vi "Write.vi"(6 "wait for reply (T)":bool=TRUE, 8 "error in (no error)":errorcluster, 10 "Command":string) -> (0 "error out":errorcluster, 1 "timed out?":bool, 2 "Reply Payload":T1)   [LabVIEW 2017, in "FingerPrintMânager.lvlib"]
doc: "_____\nCreated using Delacor QMH Event Scripter 4.1.0.80."
uses:
  Write (Reply Payload)--cluster.ctl
  Write Argument--cluster.ctl
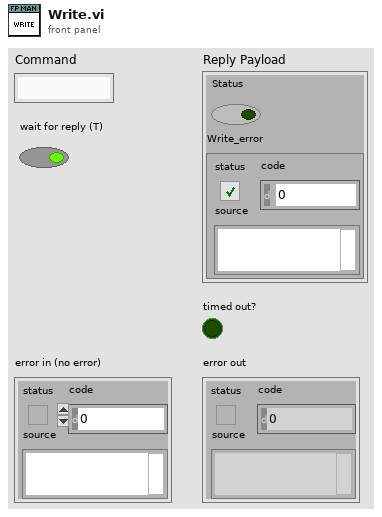
[diagram p1: front panel]
types:
  T1 = typedef "FingerPrintMânager.lvlib/Write (Reply Payload)--cluster.ctl" = cluster{"Status":bool, "Write_error":errorcluster}
  T2 = typedef "FingerPrintMânager.lvlib/Write Argument--cluster.ctl" = cluster{"Command":string, "Wait Notifier":refnum<notifier>, "wait for reply":bool}
  T3 = typedef "FingerPrintMânager.lvlib/Request Events--cluster.ctl" = cluster{"Stop Module":refnum<user-event>, "Show Panel":refnum<user-event>, "Hide Panel":refnum<user-event>, "Get Module Execution Status":refnum<user-event>, "Show Diagram":refnum<user-event>, "Init":refnum<user-event>, "UnInit":refnum<user-event>, "Write":refnum<user-event>, "Read":refnum<user-event>, "UpdatePump":refnum<user-event>, "StopPump":refnum<user-event>}
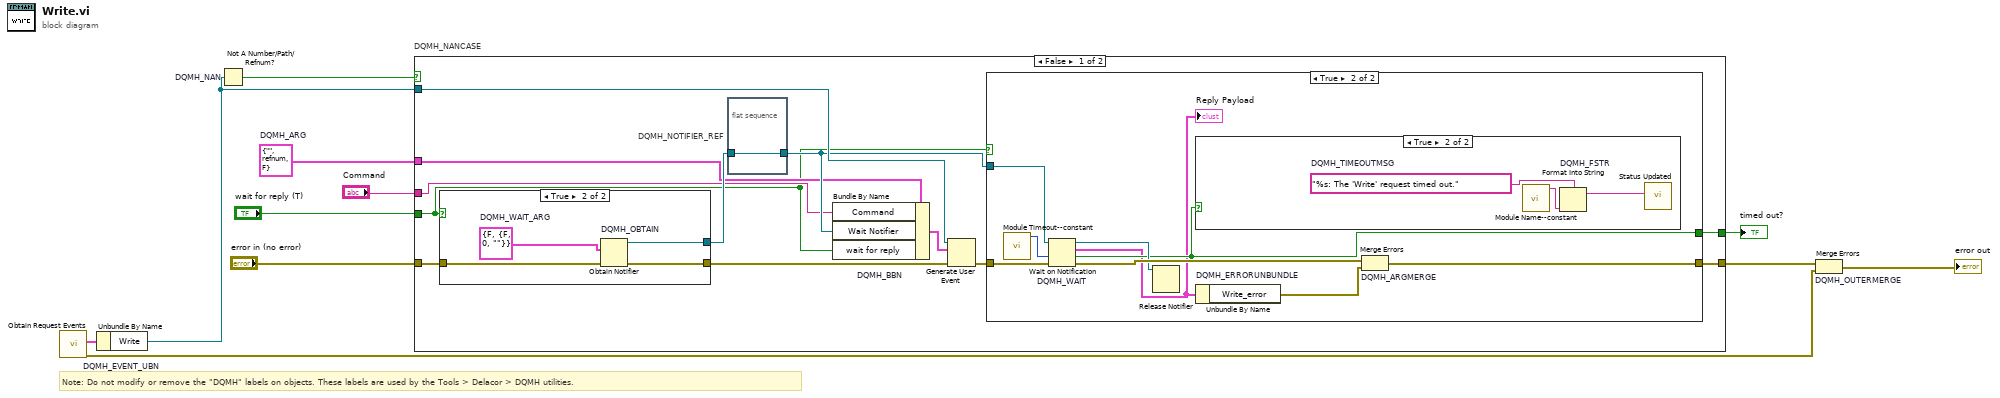
[diagram p0: block diagram]
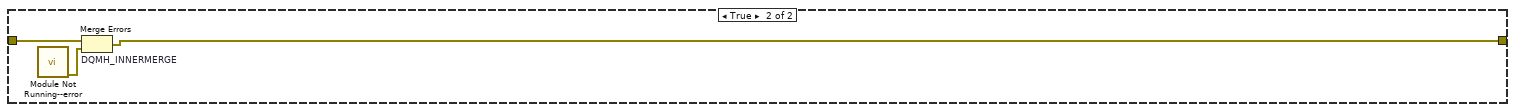
[diagram p5: hidden frame]
diagram:
  w5 = T2 {"Command"="", "Wait Notifier"=refnum, "wait for reply"=FALSE}  # DQMH_ARG
  # "Note: Do not modify or remove the \"DQMH\" labels on objects. These labels are used by the Tools > Delacor > DQMH utilities."
  n1 = call "Obtain Request Events.vi"() -> ("error out"=w2:errorcluster, "FingerPrintMânager Request Events"=w1:T3)  [unwired: 10 in]
  n2 = Unbundle By Name "DQMH_EVENT_UBN"(w1) -> ("Write"=w9:refnum<user-event>)
  n3 = Not A Number/Path/Refnum? "DQMH_NAN"(number/path/refnum=w9) -> (NaN/Path/Refnum?=w8:bool)
  n4 = case "DQMH_NANCASE" shown="False" w8 {
    tunnel: "error in (no error)" -> [w23 w45]
    tunnel: w9 -> [w21 _]
    tunnel: [w18 w44] -> w6
    tunnel: [w19 _] -> w7
    tunnel: w5 -> [w14 _]
    tunnel: "Command" -> [w13 _]
    tunnel: "wait for reply (T)" -> [w12 _]
    frame False {
      n5 = case shown="True" w12 {
        tunnel: w23 -> [w38 w42]
        tunnel: [w38 w41] -> w20
        tunnel: [_ w39] -> w16
        frame False {
        }
        frame True {
          w40 = T1 {"Status"=FALSE, "Write_error"={"status"=FALSE, "code"=0, "source"=""}}  # DQMH_WAIT_ARG
          n6 = Obtain Notifier "DQMH_OBTAIN"(notification data type=w40, error in (no error)=w42) -> (notifier out=w39:refnum<notifier>, error out=w41:errorcluster)  [unwired: 2 in, 1 out]
        }
      }
      n7 = flat-sequence "DQMH_NOTIFIER_REF" {
        tunnel: w16 -> [w24]
        tunnel: [w24] -> w15
        frame #0 {
        }
      }
      n8 = Bundle By Name "DQMH_BBN"(cluster=w14, "Command"=w13, "Wait Notifier"=w15, "wait for reply"=w12) -> (w17:T2)
      n9 = Generate User Event(user event=w21, event data cluster=w17, error in=w20) -> (error out=w22:errorcluster)  [unwired: 1 in, 1 out]
      n10 = case shown="True" w12 {
        tunnel: w22 -> [w25 w34]
        tunnel: w15 -> [_ w32]
        tunnel: [_ w30] -> w19
        tunnel: [w25 w29] -> w18
        frame False {
        }
        frame True {
          n11 = call "Module Timeout--constant.vi"() -> ("Module Timeout"=w26:i32)  [unwired: 11 in]
          n12 = Wait on Notification "DQMH_WAIT"(notifier=w32, timeout in ms (-1)=w26, error in (no error)=w34) -> (notifier out=w31:refnum<notifier>, notification=w27:T1, timed out?=w30:bool, error out=w33:errorcluster)  [unwired: 1 in]
          "Reply Payload" <- w27
          n13 = Release Notifier(notifier=w31) -> ()  [unwired: 2 in, 3 out]
          n14 = case shown="True" w30 {
            frame False {
            }
            frame True {
              w37 = "%s: The 'Write' request timed out."  # DQMH_TIMEOUTMSG
              n15 = call "Module Name--constant.vi"() -> ("Module Name"=w36:string)  [unwired: 11 in]
              n16 = Format Into String "DQMH_FSTR"(format string=w37, w36) -> (resulting string=w35:string)  [unwired: 2 in, 1 out]
              n17 = call "Status Updated.vi"("Status"=w35) -> ()  [unwired: 10 in, 1 out]
            }
          }
          n18 = Unbundle By Name "DQMH_ERRORUNBUNDLE"(w27) -> ("Write_error"=w28:errorcluster)
          n19 = Merge Errors "DQMH_ARGMERGE"(w33, w28) -> (w29:errorcluster)
        }
      }
    }
    frame True {
      n20 = call "Module Not Running--error.vi"() -> ("error out"=w43:errorcluster)  [unwired: 11 in]
      n21 = Merge Errors "DQMH_INNERMERGE"(w45, w43) -> (w44:errorcluster)
    }
  }
  "timed out?" <- w7
  n22 = Merge Errors "DQMH_OUTERMERGE"(w6, w2) -> (→"error out":errorcluster)
